vi "Get Event SubDiagram Terminals.vi"(10 "All Event Structure Tunnels":refnum<vi>[](array[refnum]), 11 "Event Subdiagram in":refnum<vi>) -> (3 "SubDiagram Terminals out":refnum<vi>[](array[refnum]))   [LabVIEW 2019, in "gRPC Template Creation Utility.lvlib"]
uses:
  gRPC Template Creation Utility.lvlib
panel:
  in  "SubDiagram Terminals":refnum<vi>[](array[refnum])
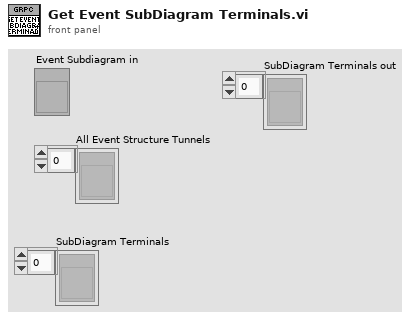
[diagram p1: front panel]
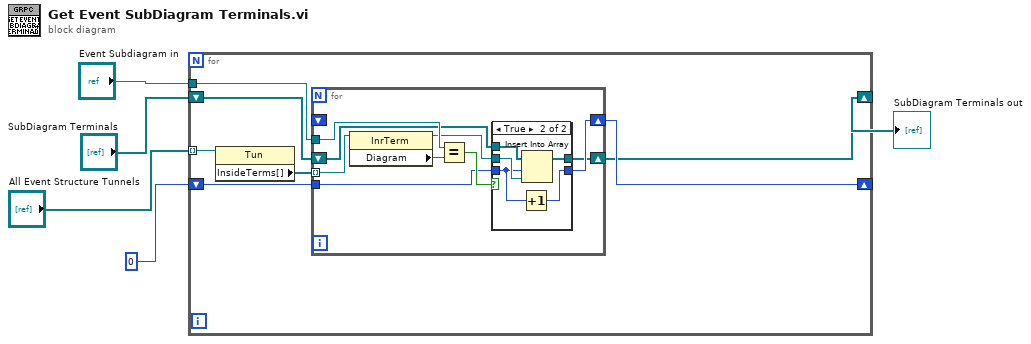
[diagram p0: block diagram]
diagram:
  n1 = for {
    tunnel: "All Event Structure Tunnels" -> [w12] mode=indexing
    tunnel: "Event Subdiagram in" -> [w10]
    shift-right: [w6] -> w1
    shift-left: "SubDiagram Terminals" -> [w9]
    shift-right: [w7] -> _
    shift-left: 0 -> [w8]
    n2 = property class="Tun"(reference=w12) -> ("InsideTerms[]"=w11:refnum<vi>[])  [unwired: 1 in, 2 out]
    n3 = for {
      tunnel: w11 -> [w21] mode=indexing
      tunnel: w10 -> [w20]
      tunnel: w8 -> [w16]
      shift-right: [w14] -> w7
      shift-left: _ -> [_]
      shift-right: [w13] -> w6
      shift-left: w9 -> [w17]
      n4 = property class="InrTerm"(reference=w21) -> (reference out=w15:refnum<vi>, "Diagram"=w19:refnum<vi>)  [unwired: 1 in, 1 out]
      n5 = Equal?(x=w20, y=w19) -> (x = y?=w18:bool)
      n6 = case shown="True" w18 {
        tunnel: w17 -> [w23 w28]
        tunnel: w16 -> [w22 w26]
        tunnel: w15 -> [_ w27]
        tunnel: [w22 w25] -> w14
        tunnel: [w23 w24] -> w13
        frame False {
        }
        frame True {
          n7 = Increment(x=w26) -> (x+1=w25:i32)
          n8 = Insert Into Array(array=w28, index=w26, new element=w27) -> (w24:refnum<vi>[])
        }
      }
    }
  }
  "SubDiagram Terminals out" <- w1
